vi "Close.vi"(8 "error in":errorcluster, 11 "Handler in":refnum<class "Handler.lvclass">) -> (0 "error out":errorcluster, 3 "Handler out":refnum<class "Handler.lvclass">)   [LabVIEW 2024, in "hse-logger.lvlib" / "Handler.lvclass"]
doc: "Tidy up any resources used by the handler. This method should be called when the ``Logger`` gets closed or the handler is removed from the ``Logger``.\n\nThis method is the implementation of the base-class and does nothing.\n\n____\nHAMPEL SOFTWARE ENGINEERING v2.2.2 (2025-01-16 15:41)"
uses:
  <vilib>/Hampel Software Engineering/HSE Logger/Handler/Handler.lvclass
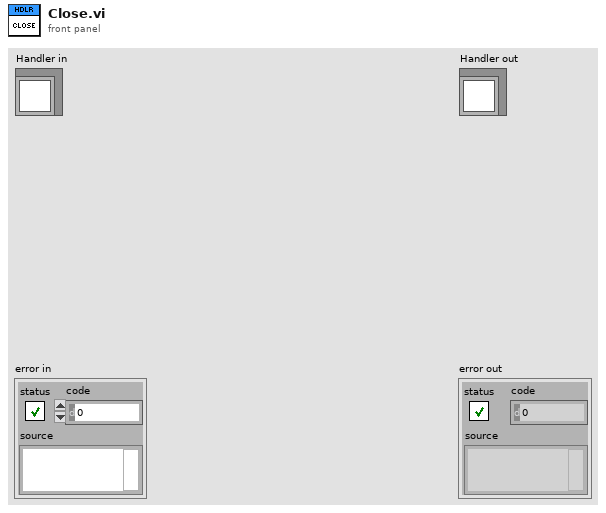
[diagram p1: front panel]
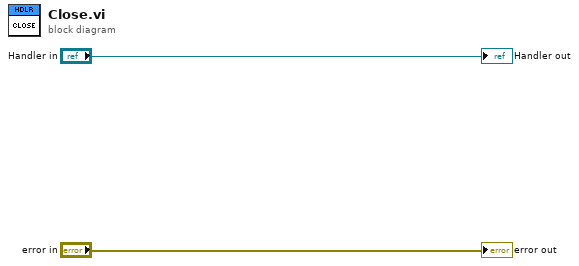
[diagram p0: block diagram]
diagram:
  "error out" <- "error in"
  "Handler out" <- "Handler in"
